vi "temp.vi"() -> ()   [LabVIEW 2013]
panel:
  out "output 16":bool
  out "output 15":bool
  out "output 14":dbl
  out "output 13":dbl
  out "output 12":dbl
  out "output 11":dbl
  out "output 10":dbl
  out "output 9":dbl
  out "s4":string
  out "output 8":dbl
  out "s3":string
  out "output 7":dbl
  out "s2":string
  out "output 6":dbl
  out "s1":string
  out "output 5":dbl
  in  "format string 2":string
  in  "format string":string
  in  "input string 3":string
  in  "input string 2":string
  out "selection":bool
  out "output string":string
  in  "true string":string
  out "output 4":i32
  out "output 3":i32
  out "output 2":dbl
  out "output 1":u8
  out "remaining string":string
  in  "input string":string
  out "element":string
  in  "thcd_com 2":T1(ring)
  out "resulting string 2":string
  in  "input 1":dbl min=0.0 max=250.0 step=2.0 format="%#.6g"
  out "resulting string":string
  in  "thcd_ch":u8
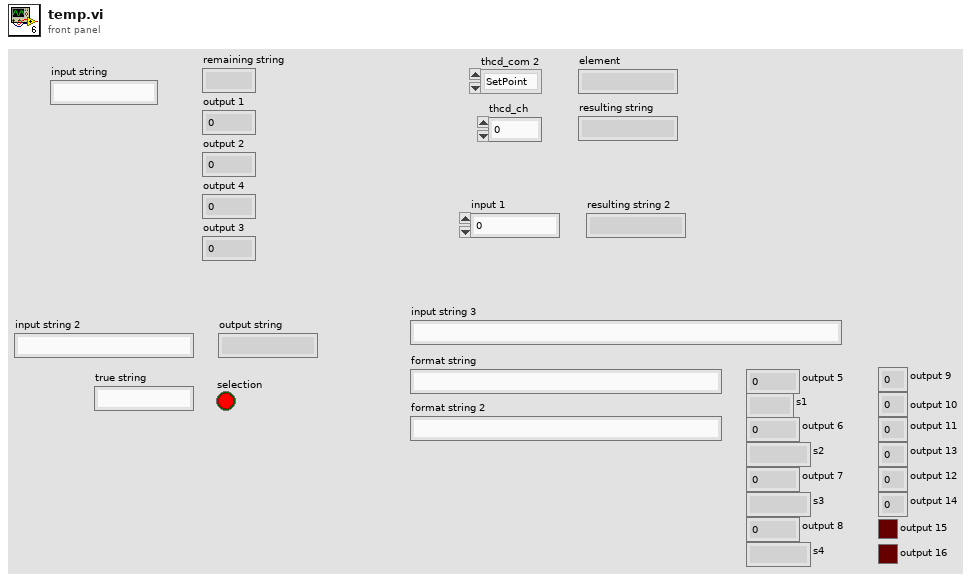
[diagram p1: front panel]
types:
  T1 = enum16{"SetPoint", "AlarmH", "AlarmL", "AlarmHys", "Units", "GasID", "SigInput", "Filter", "Multiplier", "Display", "ReadCh"}
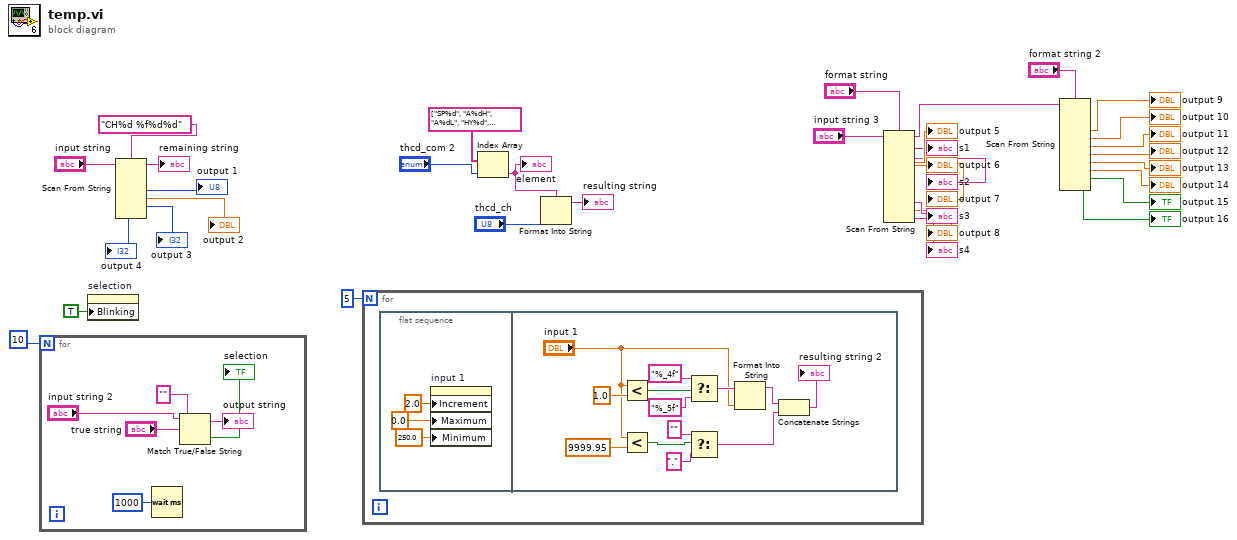
[diagram p0: block diagram]
diagram:
  n1 = for {
    N: 10 -> [_]
    n2 = Wait (ms)(milliseconds to wait=u32 1000) -> ()  [unwired: 1 out]
    n3 = Match True/False String(2:"" ("false string"), 3:"true string", 4:"input string 2") -> (0:→"selection":bool, 1:→"output string":string)
  }
  n4 = property on="selection" class="Bool (strict)"("Blinking"=TRUE) -> ()  [unwired: 2 in, 2 out]
  n5 = Scan From String(format string="CH%d %f%d%d" ("string"), input string="input string") -> (remaining string=→"remaining string":string, output 1=→"output 1":u8, output 2=→"output 2":dbl, output 3=→"output 3":i32, output 4=→"output 4":i32)  [unwired: 6 in, 2 out]
  n6 = for {
    N: 5 -> [_]
    n7 = flat-sequence {
      frame #0 {
        n8 = property on="input 1" class="DigNum (strict)"("Increment"=2.0 ("Data Entry Limits:Increment"), "Maximum"=0.0 ("Data Entry Limits:Maximum"), "Minimum"=250.0 ("Data Entry Limits:Minimum")) -> ()  [unwired: 2 in, 2 out]
      }
      frame #1 {
        n9 = Less?(x="input 1", y=1.0) -> (x < y?=w54:bool)
        n10 = Less?(x="input 1", y=9999.95) -> (x < y?=w46:bool)
        n11 = Select(t="%_4f" ("format string"), s=w54, f="%_5f" ("format string")) -> (s? t:f=w53:string)
        n12 = Select(t="" ("format string"), s=w46, f="." ("format string")) -> (s? t:f=w45:string)
        n13 = Format Into String(format string=w53, "input 1") -> (resulting string=w52:string)  [unwired: 2 in, 1 out]
        n14 = Concatenate Strings(w52, w45) -> (→"resulting string 2":string)
      }
    }
  }
  n15 = Index Array(array=string[] ["SP%d", "A%dH", "A%dL", "HY%d", "UM%d", "GS%d", "IN%d", "FL%d", "ML%d", "D%d", "C%d"] ("Array"), index="thcd_com 2") -> (element=w33:string)
  "element" <- w33
  n16 = Format Into String(format string=w33, "thcd_ch") -> (resulting string=→"resulting string":string)  [unwired: 2 in, 1 out]
  n17 = Scan From String(format string="format string", input string="input string 3") -> (remaining string=w11:string, output 1=→"output 5":dbl, output 2=→"s1":string, output 3=→"output 6":dbl, output 4=→"s2":string, output 5=→"output 7":dbl, output 6=→"s3":string, output 7=→"output 8":dbl, output 8=→"s4":string)  [unwired: 10 in, 2 out]
  n18 = Scan From String(format string="format string 2", input string=w11) -> (output 1=→"output 9":dbl, output 2=→"output 10":dbl, output 3=→"output 11":dbl, output 4=→"output 12":dbl, output 5=→"output 13":dbl, output 6=→"output 14":dbl, output 7=→"output 15":bool, output 8=→"output 16":bool)  [unwired: 10 in, 3 out]
